vi "SetCtlValueSGNL_Core.vi"(8 "error in (no error)":errorcluster, 9 "Value":variant, 10 "CtlName In":string, 11 "ctlRef_Maps in":refnum<class "ctlRef_Maps.lvclass">) -> (0 "error out":errorcluster, 3 "ctlRef_Maps out":refnum<class "ctlRef_Maps.lvclass">)   [LabVIEW 2020, in "CtlReferences.lvlib" / "ctlRef_Maps.lvclass"]
uses:
  ctlRef_Maps.lvclass
  ctlRef_Maps.lvclass/ctlRef_Maps.ctl
  CtlReferences/CtlReferences.lvclass
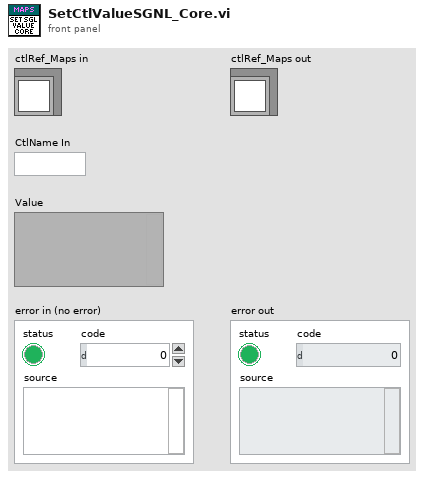
[diagram p1: front panel]
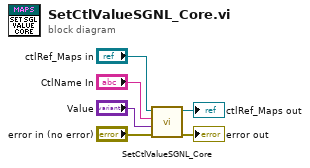
[diagram p0: block diagram]
diagram:
  n1 = call-parent "SetCtlValueSGNL_Core.vi"("error in (no error)"="error in (no error)", "Value"="Value", "CtlName In"="CtlName In", "CtlReferences in"="ctlRef_Maps in") -> ("error out"=→"error out":errorcluster, "CtlReferences out"=→"ctlRef_Maps out":refnum<class "ctlRef_Maps.lvclass">)  [unwired: 6 in]
